vi "project.vi"() -> ()   [LabVIEW 2022 SP3]
panel:
  in  "Enum":enum16{"farenheit", "celsius", "kelvin"}(ring)
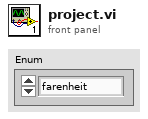
[diagram p1: front panel]
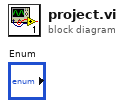
[diagram p0: block diagram]
diagram:
